vi "Bounds - thread count.vi"(8 "error in (no error)":errorcluster) -> (0 "error out":errorcluster, 1 "max_count":i32, 2 "min_count":i32)   [LabVIEW 2020, in "lvzstd.lvlib"]
uses:
  lvzstd.lvlib
  Private/Path FGV.vi
  <vilib>/Utility/error.llb/Error Cluster From Error Code.vi
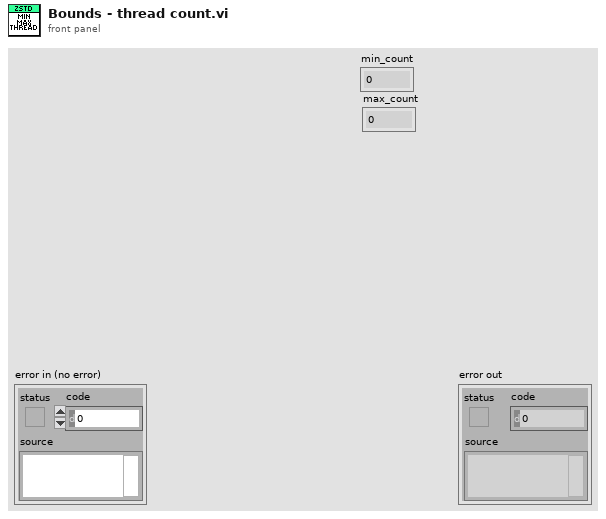
[diagram p1: front panel]
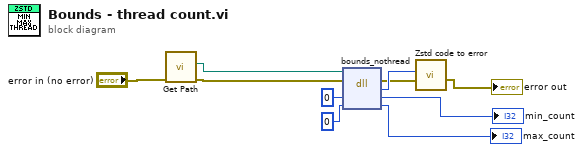
[diagram p0: block diagram]
diagram:
  n1 = call "Get Path.vi"("error in (no error)"="error in (no error)") -> ("error out (no error)"=w2:errorcluster, "Library Path"=w1:path)  [unwired: 9 in]
  n2 = dll-call lib="?" fn="bounds_nothread"(path in=w1, error in=w2, "min_count"=0, "max_count"=0 ("max_compressed_size")) -> (error out=w5:errorcluster, "return type"=w6:i32, "min_count"=→"min_count":i32, "max_count"=→"max_count":i32)  [unwired: 1 in, 1 out]
  n3 = call "Zstd code to error.vi"("error in"=w5, "Error code"=w6) -> ("error in (no error)"=→"error out":errorcluster)  [unwired: 9 in]
